vi "Display.vi"(8 "error in":errorcluster, 11 "Custom - Timeout in":refnum<class "Gif - Timeout.lvclass">) -> (0 "error out":errorcluster, 3 "Custom - Timeout out":refnum<class "Gif - Timeout.lvclass">)   [LabVIEW 2021, in "Gif - Timeout.lvclass"]
doc: "This vi displays the custom timeout Popup.\n\n<b>Code Developed By:</b>\nDaniel Coons\nTechnology Service Corporation\n1983 S Liberty Drive\nBloomington, IN 47403\nPhone: 812 558-7100\ndaniel.coons@tsc.com\nwww.tsc.com/atcs"
uses:
  Gif - Timeout.lvclass
  C:/Program Files/National Instruments/LabVIEW 2024/vi.lib/addons/_TSC/TSC Pop-Up/Popup/Popup.lvclass
  C:/Development/tsc-pop-up-gif/GIF Parent.lvclass
  <vilib>/Utility/miscctls.llb/LVPositionTypeDef.ctl
  <vilib>/addons/_TSC/TSC Pop-Up/Popup/Popup.lvclass/Popup.ctl
  GIF Parent.lvclass/GIF Parent.ctl
  Gif - Timeout.lvclass/Gif - Timeout.ctl
  <vilib>/addons/_TSC/TSC Pop-Up/Popup/Data Member Access/Read Theme.vi
  Read Delays.vi
  Read Gif Images.vi
  <vilib>/addons/_TSC/TSC Pop-Up/Theme/Theme.lvclass
  <vilib>/addons/_TSC/TSC Pop-Up/Popup/Popup.lvclass
  user32.dll
panel:
  in  "closer":bool
  out "header":bool
  out "count":string
  out "2D Picture":picture
  out "Message":string
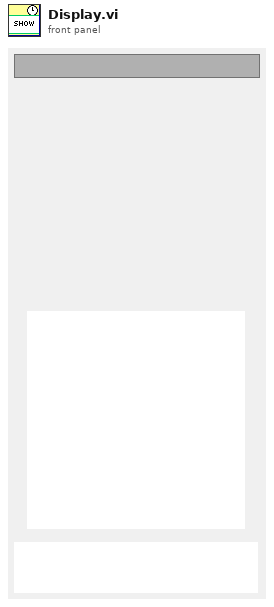
[diagram p1: front panel]
types:
  T1 = typedef "LVPositionTypeDef.ctl" = cluster{"Left":i32, "Top":i32}
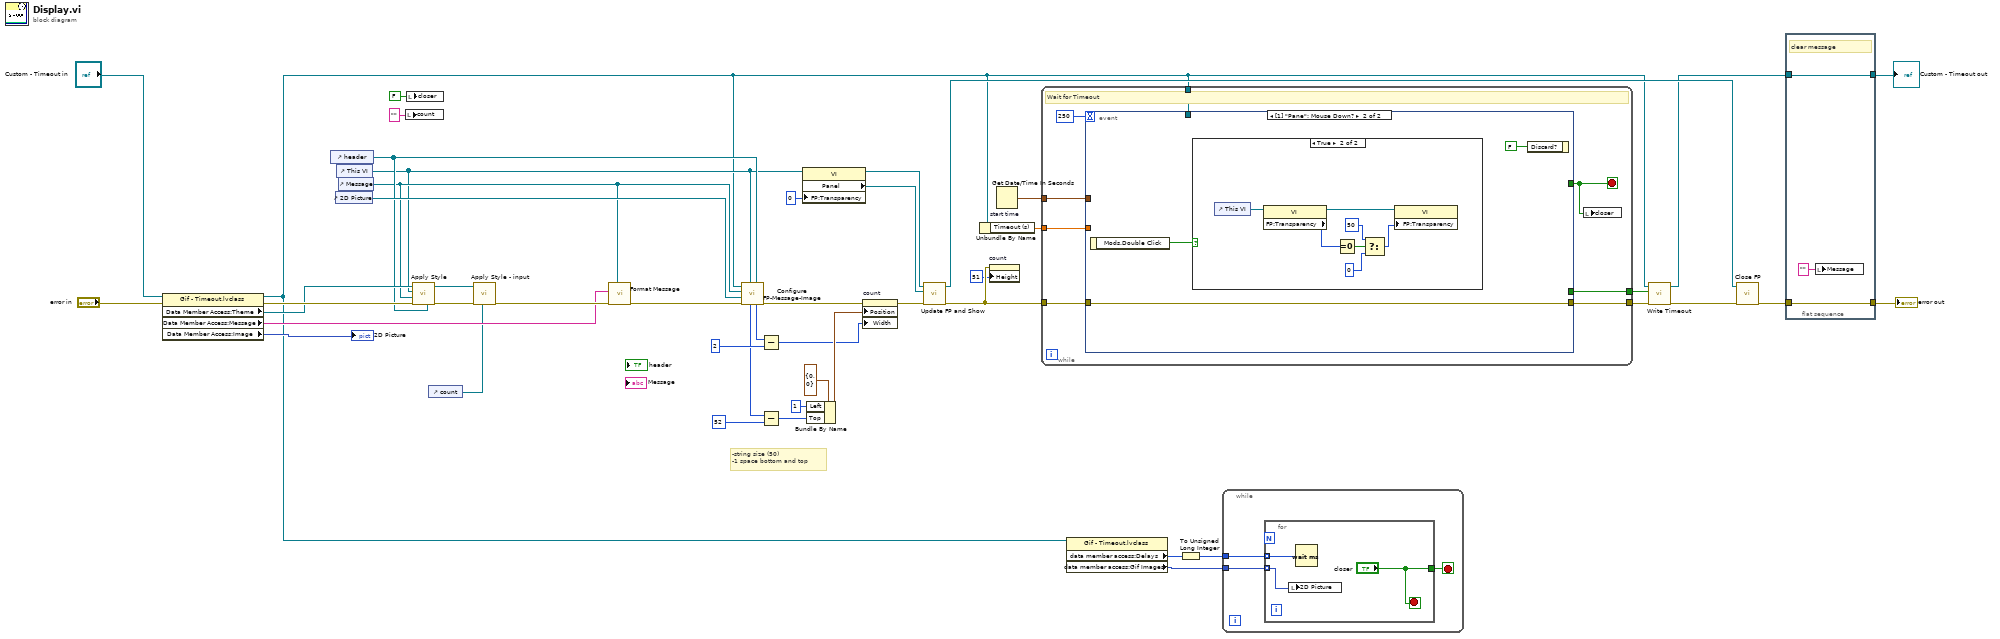
[diagram p0: block diagram]
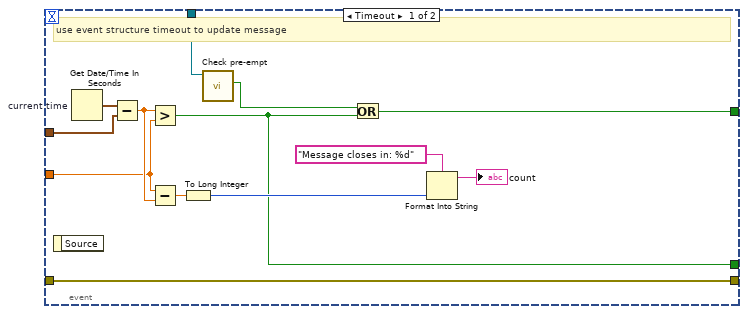
[diagram p2: hidden frame]
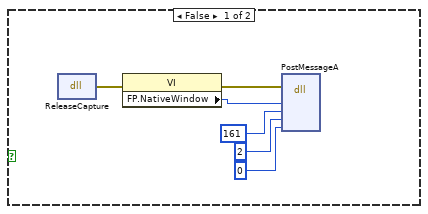
[diagram p3: hidden frame]
diagram:
  # "-string size (50)\n-1 space bottom and top"
  n1 = property class="Gif - Timeout.lvclass"(reference="Custom - Timeout in", error in="error in") -> (reference out=w3:refnum<class "Gif - Timeout.lvclass">, error out=w31:errorcluster, "Data Member Access:Theme"=w30:refnum<class "Theme.lvclass">, "Data Member Access:Message"=w16:string, "Data Member Access:Image"=→"2D Picture":picture)
  n2 = control-ref of="header"() -> (w20:refnum<vi>)
  n3 = control-ref of="2D Picture"() -> (w27:refnum<vi>)
  n4 = control-ref of="This VI"() -> (w14:refnum<vi>)
  n5 = control-ref of="Message"() -> (w19:refnum<vi>)
  n6 = local write "count"("" ("count")) -> ()
  n7 = local write "closer"(FALSE ("closer")) -> ()
  n8 = call <vilib>:"Apply Style.vi"("header ref"=w20, "error in (no error)"=w31, "message ref"=w19, "pop up ref"=w14, "Theme in"=w30) -> ("error out"=w21:errorcluster, "Theme out"=w17:refnum<class "Theme.lvclass">)  [unwired: 5 in]
  n9 = control-ref of="count"() -> (w15:refnum<vi>)
  n10 = call <vilib>:"Apply Style - input.vi"("input ref"=w15, "error in (no error)"=w21, "Theme in"=w17) -> ("error out"=w18:errorcluster)  [unwired: 7 in, 1 out]
  n11 = call <vilib>:"Format Message.vi"("formatted string"=w19, "error in"=w18, "String Input"=w16) -> ("error out"=w29:errorcluster)  [unwired: 7 in, 1 out]
  n12 = call <vilib>:"Configure FP-Message-Image.vi"("header ref"=w20, "Pop Up ref"=w14, "error in (no error)"=w29, "Image ref"=w27, "Message ref"=w19, "Popup in"=w3) -> ("error out"=w28:errorcluster, "Panel Width"=w24:i32, "Panel Height"=w22:i32)  [unwired: 1 in, 2 out]
  n13 = Subtract(x=w24, y=2) -> (x-y=w23:i32)
  n14 = Subtract(x=w22, y=52) -> (x-y=w35:i32)
  n15 = property class="VI"(reference=w14, "FP:Transparency"=u8 0 ("Front Panel Window:Transparency")) -> (reference out=w13:refnum<vi>, "Panel"=w12:refnum<vi>)  [unwired: 1 in, 1 out]
  n16 = Bundle By Name(cluster=T1 {"Left"=0, "Top"=0} ("Position"), "Left"=1, "Top"=w35) -> (w34:T1)
  n17 = property on="count" class="Str"(error in=w28, "Position"=w34, "Width"=w23) -> (error out=w26:errorcluster)  [unwired: 1 in, 1 out]
  n18 = call <vilib>:"Update FP and Show.vi"("error in (no error)"=w26, "Panel Ref"=w12, "VI in"=w13) -> ("error out"=w10:errorcluster, "VI out"=w41:refnum<vi>)  [unwired: 7 in]
  n19 = Unbundle By Name(w3) -> ("Timeout (s)"=w45:dbl)
  n20 = property on="count" class="Str"(error in=w10, "Height"=u32 51 ("Size:Height")) -> ()  [unwired: 1 in, 2 out]
  n21 = Get Date/Time In Seconds "start time"() -> (seconds since 1Jan1904=w46:timestamp)
  n22 = while {
    tunnel: [w51] -> w47
    tunnel: w10 -> [w52]
    tunnel: w46 -> [w55]
    tunnel: w45 -> [w54]
    tunnel: w3 -> [w50]
    tunnel: [w48] -> w1
    stop <- w49 stop-if-true
    # "Wait for Timeout"
    n23 = event shown="[1] \"Pane\": Mouse Down?" {
      selector: _ -> [_ _]
      dyn-events: _ -> [_ _]
      timeout: 250 -> [_ _]
      tunnel: w55 -> [w68 _]
      tunnel: [w60 _] -> w49
      tunnel: w54 -> [w64 _]
      tunnel: w52 -> [w61 w70]
      tunnel: [w61 w70] -> w51
      tunnel: w50 -> [w58 _]
      tunnel: [w56 _] -> w48
      event Timeout {
        # "use event structure timeout to update message"
        n24 = event-data() -> ()  [unwired: 1 in, 1 out]
        n25 = Get Date/Time In Seconds "current time"() -> (seconds since 1Jan1904=w67:timestamp)
        n26 = Subtract(x=w67, y=w68) -> (x-y=w66:dbl)
        n27 = Greater?(x=w66, y=w64) -> (0:w56:bool)
        n28 = Subtract(x=w64, y=w66) -> (x-y=w65:dbl)
        n29 = To Long Integer(number=w65) -> (32bit integer=w62:i32)
        n30 = call <vilib>:"Check pre-empt.vi"("_Popup in"=w58) -> ("Pre-empted?"=w59:bool)  [unwired: 8 in, 2 out]
        n31 = Or(x=w59, y=w56) -> (x .or. y?=w60:bool)
        n32 = Format Into String(format string="Message closes in: %d", w62) -> (resulting string=→"count":string)  [unwired: 2 in, 1 out]
      }
      event Mouse Down? {
        n33 = event-data() -> ("Mods.Double Click"=w69:bool)  [unwired: 1 in]
        n34 = case shown="True" w69 {
          frame False {
            n35 = dll-call lib="user32.dll" fn="ReleaseCapture"() -> (error out=w75:errorcluster)  [unwired: 4 in, 1 out]
            n36 = property class="VI"(error in=w75) -> (error out=w76:errorcluster, "FP.NativeWindow"=w77:u64)  [unwired: 1 in, 1 out]
            n37 = dll-call lib="user32.dll" fn="PostMessageA"(error in=w76, "hWnd"=w77, "Msg"=161, "wParam"=2, "lParam"=0) -> ()  [unwired: 7 in, 2 out]
          }
          frame True {
            n38 = control-ref of="This VI"() -> (w84:refnum<vi>)
            n39 = property class="VI"(reference=w84) -> (reference out=w82:refnum<vi>, "FP:Transparency"=w83:u8)  [unwired: 1 in, 1 out]
            n40 = Equal To 0?(x=w83) -> (x = 0?=w81:bool)
            n41 = Select(t=u8 50, s=w81, f=u8 0) -> (s? t:f=w80:u8)
            n42 = property class="VI"(reference=w82, "FP:Transparency"=w80) -> ()  [unwired: 1 in, 2 out]
          }
        }
        n43 = event-data("Discard?"=FALSE) -> ()  [unwired: 1 in, 1 out]
      }
    }
    n44 = local write "closer"(w49) -> ()
  }
  n45 = property class="Gif - Timeout.lvclass"(reference=w3) -> ("data member access:Delays"=w8:i32[], "data member access:Gif Images"=w7:picture[])  [unwired: 1 in, 2 out]
  n46 = To Unsigned Long Integer(number=w8) -> (unsigned 32bit integer=w6:u32[])
  n47 = while {
    tunnel: w6 -> [w86]
    tunnel: w7 -> [w85]
    stop <- w87 stop-if-true
    n48 = for {
      tunnel: ["closer"] -> w87
      tunnel: w86 -> [w89] mode=indexing
      tunnel: w85 -> [w88] mode=indexing
      stop <- "closer" stop-if-true
      n49 = local write "2D Picture"(w88) -> ()
      n50 = Wait (ms)(milliseconds to wait=w89) -> ()  [unwired: 1 out]
    }
  }
  n51 = call <vilib>:"Write Timeout.vi"("error in (no error)"=w47, "Timeout?"=w1, "Popup in"=w3) -> ("error out"=w4:errorcluster, "Popup out"=w2:refnum<class "Gif - Timeout.lvclass">)  [unwired: 7 in]
  n52 = call <vilib>:"Close FP.vi"("error in (no error)"=w4, "VI in"=w41) -> ("error out"=w40:errorcluster)  [unwired: 9 in]
  n53 = flat-sequence {
    tunnel: w40 -> [w93]
    tunnel: [w93] -> w39
    tunnel: w2 -> [w92]
    tunnel: [w92] -> w38
    frame #0 {
      # "clear message"
      n54 = local write "Message"("" ("Message")) -> ()
    }
  }
  "error out" <- w39
  "Custom - Timeout out" <- w38
